vi "Teardown Created Queues.vi"(11 "Base Queue in":refnum<class "Base Queue.lvclass">) -> (3 "Base Queue out":refnum<class "Base Queue.lvclass">)   [LabVIEW 2021, in "jettl.lvlib" / "Base Queue.lvlib" / "Base Queue.lvclass"]
uses:
  Base Queue.lvclass
  jettl Msg Teardown/jettl Msg Teardown.lvlib
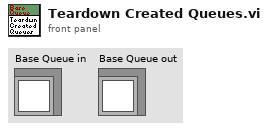
[diagram p1: front panel]
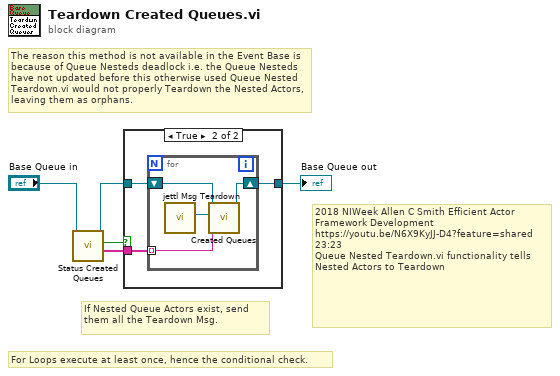
[diagram p0: block diagram]
diagram:
  # "2018 NIWeek Allen C Smith Efficient Actor Framework Development\nhttps://youtu.be/N6X9KyJJ-D4?feature=shared\n23:23\nQueue Nested Teardown.vi functionality tells Nested Actors to Teardown"
  # "For Loops execute at least once, hence the conditional check."
  # "If Nested Queue Actors exist, send them all the Teardown Msg."
  # "The reason this method is not available in the Event Base is because of Queue Nesteds deadlock i.e. the Queue Nesteds have not updated before this otherwise used Queue Nested Teardown.vi would not properly Teardown the Nested Actors, leaving them as orphans."
  n1 = call-dynamic "Status Created Queues.vi"("Base Queue in"="Base Queue in") -> ("Created Queue Aliases"=w1:string[], "Created Queue Exist?"=w2:bool, "Base Queue out"=w3:refnum<class "Base Queue.lvclass">)  [unwired: 7 in, 1 out]
  n2 = case shown="True" w2 {
    tunnel: [w6 w9] -> w5
    tunnel: w3 -> [w6 w8]
    tunnel: w1 -> [_ w7]
    frame False {
    }
    frame True {
      n3 = for {
        tunnel: w7 -> [w13] mode=indexing
        shift-right: [w11] -> w9
        shift-left: w8 -> [w12]
        n4 = call "jettl Msg Teardown.vi"() -> ("Msg Strategy"=w10:refnum<class "Msg Strategy.lvclass">)  [unwired: 11 in]
        n5 = call-dynamic "Created Queues.vi"("Created Queue Alias"=w13, "Msg Strategy"=w10, "Base Queue in"=w12) -> ("Base Queue out"=w11:refnum<class "Base Queue.lvclass">)  [unwired: 8 in]
      }
    }
  }
  "Base Queue out" <- w5
